vi "App_Registering.vi"(8 "error in":errorcluster, 11 "Registering Data":T2) -> (0 "error out":errorcluster)   [LabVIEW 2015, in "Application 1.lvlib"]
uses:
  Application 1.lvlib
  <vilib>/vision/Image Controls.llb/IMAQ Image.ctl
  Com VIs/Data Def/User Data.ctl
  Com VIs/Data Def/User Registering Status.ctl
  Data Def/App_Main Loop Queue Data.ctl
  Data Def/App_Subpanel Name.ctl
  Data Def/App_User Event Data.ctl
  Data Def/App_Config Method.ctl
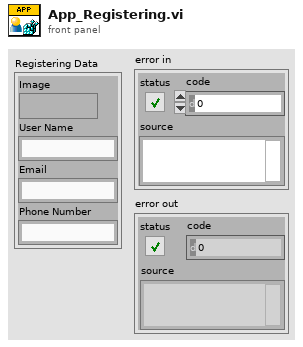
[diagram p1: front panel]
types:
  T1 = typedef "IMAQ Image.ctl" = refnum<image>
  T2 = cluster{"Image":T1, "User Name":string, "Email":string, "Phone Number":string}
  T3 = typedef "User Data.ctl" = cluster{"Name":string, "Email":string, "Phone Number":string, "User Picture":u32[][], "Last Login Time":timestamp}
  T4 = typedef "Application 1.lvlib/App_User Event Data.ctl" = cluster{"Command":string, "Data":variant}
  T5 = typedef "Application 1.lvlib/App_Subpanel Name.ctl" = enum16{"Main", "Menu", "User Registering", "User Setting", "Monitor", "Traning Mode", "Query Data", "Connect Setting"}
  T6 = typedef "Application 1.lvlib/App_Config Method.ctl" = enum16{"Get", "Put", "Load", "Save"}
  T7 = typedef "Application 1.lvlib/App_Main Loop Queue Data.ctl" = cluster{"Command":string, "Data":variant}
  T8 = typedef "User Registering Status.ctl" = enum16{"Failed", "Duplicate", "Success"}
  T9 = typedef "Application 1.lvlib/App_Main Data.ctl" = cluster{"VI Refnum":refnum<vi>, "Subpanel":refnum<vi>, "Connection ID":refnum<k5>, "Meta data":T10[], "Main Queue":T12, "User Data":T3}
  T10 = typedef "stm_MetaElement.ctl" = cluster{"Name":T11}
  T11 = typedef "stm_MetaDataElement.ctl" = string
  T12 = typedef "Application 1.lvlib/App_Main Queue.ctl" = cluster{"Main Loop Queue":refnum<queue>}
  T13 = typedef "Application 1.lvlib/App_Configuration.ctl" = cluster{"Server IP":string, "User Name":string}
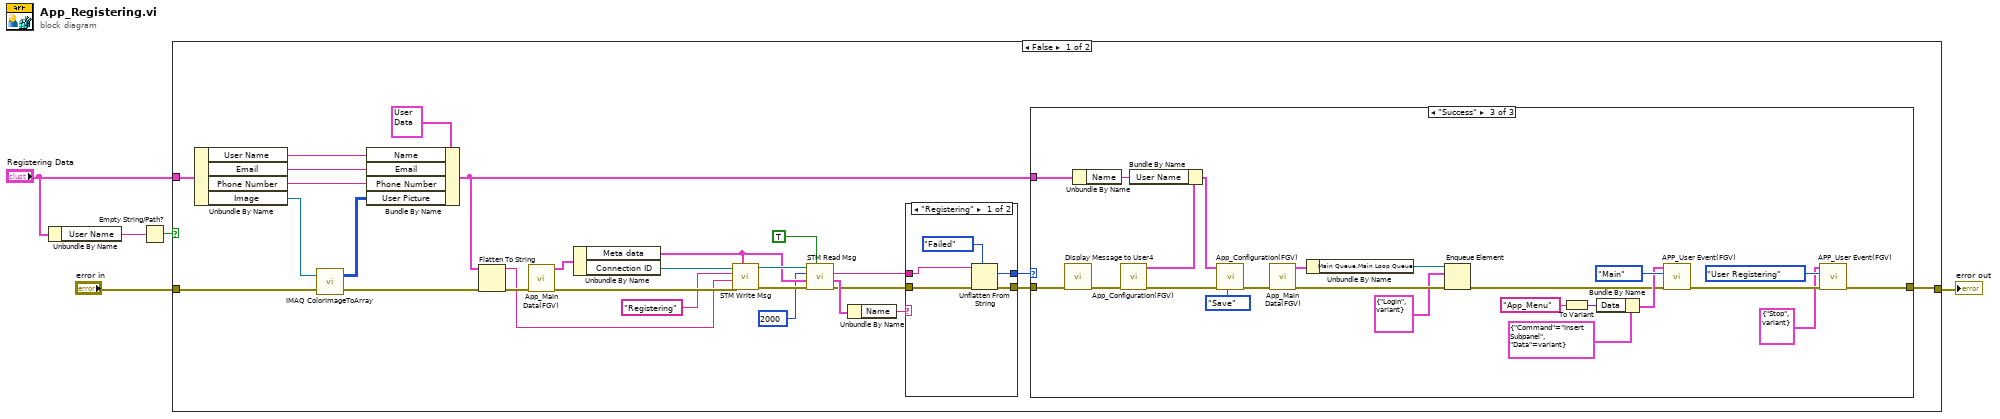
[diagram p0: block diagram]
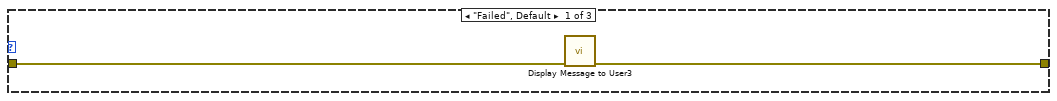
[diagram p2: hidden frame]
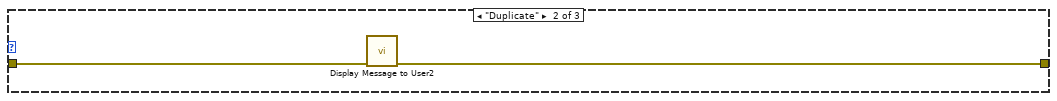
[diagram p3: hidden frame]
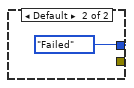
[diagram p4: hidden frame]
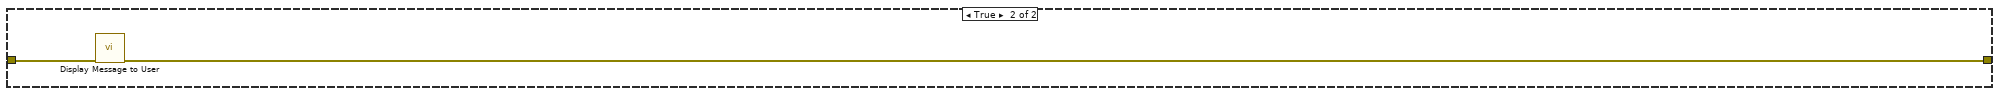
[diagram p5: hidden frame]
diagram:
  n1 = Unbundle By Name("Registering Data") -> ("User Name"=w5:string)
  n2 = Empty String/Path?(string/path=w5) -> (empty?=w4:bool)
  n3 = case shown="False" w4 {
    tunnel: "Registering Data" -> [w33 _]
    tunnel: "error in" -> [w32 w68]
    tunnel: [w8 w67] -> w1
    frame False {
      n4 = Unbundle By Name(w33) -> ("User Name"=w29:string, "Email"=w28:string, "Phone Number"=w27:string, "Image"=w31:T1)
      n5 = call "IMAQ ColorImageToArray"("Image"=w31, "error in (no error)"=w32) -> ("Image Pixels (U32)"=w26:u32[][], "error out"=w21:errorcluster)  [unwired: 2 in, 1 out]
      n6 = Bundle By Name(cluster=T3 {"Name"="Guset", "Email"="", "Phone Number"="", "User Picture"=array225x225[50625 elements], "Last Login Time"=timestamp(0 s since 1904-01-01)} ("User Data"), "Name"=w29, "Email"=w28, "Phone Number"=w27, "User Picture"=w26) -> (w7:T3)
      n7 = Flatten To String(anything=w7, error in (no error)=w21) -> (data string=w19:string, error out=w20:errorcluster)  [unwired: 2 in, 1 out]
      n8 = call "App_Main Data(FGV).vi"("error in"=w20) -> ("error out"=w24:errorcluster, "Main Data Out"=w25:T9)  [unwired: 9 in]
      n9 = Unbundle By Name(w25) -> ("Meta data"=w16:T10[], "Connection ID"=w23:refnum<k5>)
      n10 = call "STM Write Msg.vi"("Meta data"=w16, "error in (no error)"=w24, "Data"=w19, "Name"="Registering", "connection ID"=w23) -> ("error out"=w18:errorcluster, "connection ID out"=w17:refnum<k5>)  [unwired: 5 in]
      n11 = call "STM Read Msg.vi"("Ignore Timeout Error"=TRUE, "error in"=w18, "Meta data"=w16, "timeout ms (25000)"=2000, "connection ID"=w17) -> ("error out"=w12:errorcluster, "Meta element"=w14:T10, "data string"=w11:string)  [unwired: 1 in, 3 out]
      n12 = Unbundle By Name(w14) -> ("Name"=w13:T11)
      n13 = case shown="\"Registering\"" w13 {
        tunnel: w12 -> [w65 _]
        tunnel: w11 -> [w64 _]
        tunnel: [w62 User_Registering_Status."Failed" ("User Registering Status")] -> w10
        tunnel: [w61 _] -> w9
        frame "Registering" {
          n14 = Unflatten From String(type=User_Registering_Status."Failed" ("User Registering Status"), binary string=w64, error in (no error)=w65) -> (value=w62:T8, error out=w61:errorcluster)  [unwired: 2 in, 1 out]
        }
        frame Default {
        }
      }
      n15 = case shown="\"Success\"" w10 {
        tunnel: w9 -> [w35 w37 w60]
        tunnel: [w34 w36 w39] -> w8
        tunnel: w7 -> [_ _ w48]
        frame "Failed", Default {
          n16 = call "Display Message to User3"("error in (no error)"=w35) -> ("error out"=w34:errorcluster)  [unwired: 9 in, 1 out]
        }
        frame "Duplicate" {
          n17 = call "Display Message to User2"("error in (no error)"=w37) -> ("error out"=w36:errorcluster)  [unwired: 9 in, 1 out]
        }
        frame "Success" {
          n18 = call "Display Message to User4"("error in (no error)"=w60) -> ("error out"=w49:errorcluster)  [unwired: 9 in, 1 out]
          n19 = Unbundle By Name(w48) -> ("Name"=w46:string)
          n20 = call "App_Configuration(FGV).vi"("error in"=w49) -> ("error out"=w45:errorcluster, "Configuration Out"=w47:T13)  [unwired: 9 in]
          n21 = Bundle By Name(cluster=w47, "User Name"=w46) -> (w44:T13)
          n22 = call "App_Configuration(FGV).vi"("Config Method(Get)"=App_Config_Method."Save", "error in"=w45, "Configuration In"=w44) -> ("error out"=w42:errorcluster)  [unwired: 7 in, 1 out]
          n23 = call "App_Main Data(FGV).vi"("error in"=w42) -> ("error out"=w58:errorcluster, "Main Data Out"=w59:T9)  [unwired: 9 in]
          n24 = Unbundle By Name(w59) -> ("Main Queue.Main Loop Queue"=w57:refnum<queue>)
          n25 = Enqueue Element(queue=w57, element=T7 {"Command"="Login", "Data"=variant}, error in (no error)=w58) -> (error out=w50:errorcluster)  [unwired: 1 in, 2 out]
          n26 = To Variant(anything="App_Menu") -> (Variant=w53:variant)
          n27 = Bundle By Name(cluster=T4 {"Command"="Insert Subpanel", "Data"=variant} ("User Event Data"), "Data"=w53) -> (w51:T4)
          n28 = call "APP_User Event(FGV).vi"("error in"=w50, "Subpanel Name"=App_Subpanel_Name."Main", "User Event Data"=w51) -> ("error out"=w41:errorcluster)  [unwired: 7 in, 1 out]
          n29 = call "APP_User Event(FGV).vi"("error in"=w41, "Subpanel Name"=App_Subpanel_Name."User Registering", "User Event Data"=T4 {"Command"="Stop", "Data"=variant}) -> ("error out"=w39:errorcluster)  [unwired: 7 in, 1 out]
        }
      }
    }
    frame True {
      n30 = call "Display Message to User"("error in (no error)"=w68) -> ("error out"=w67:errorcluster)  [unwired: 9 in, 1 out]
    }
  }
  "error out" <- w1
